vi "Read older Metadata channels.vi"(1 "Number of Channels":i32) -> (0 "Initial Info Cluster":T1[](array[typedef]))   [LabVIEW 2022 SP3]
uses:
  Controls/Initial Info Cluster.ctl
  Globals/Meas_global.vi
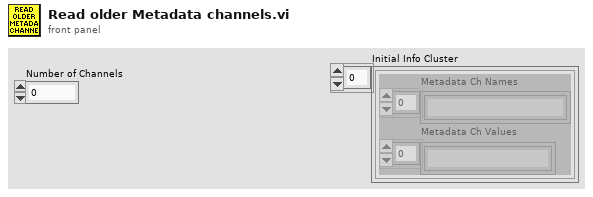
[diagram p1: front panel]
types:
  T1 = typedef "Initial Info Cluster.ctl" = cluster{"Metadata Ch Names":string[], "Metadata Ch Values":string[]}
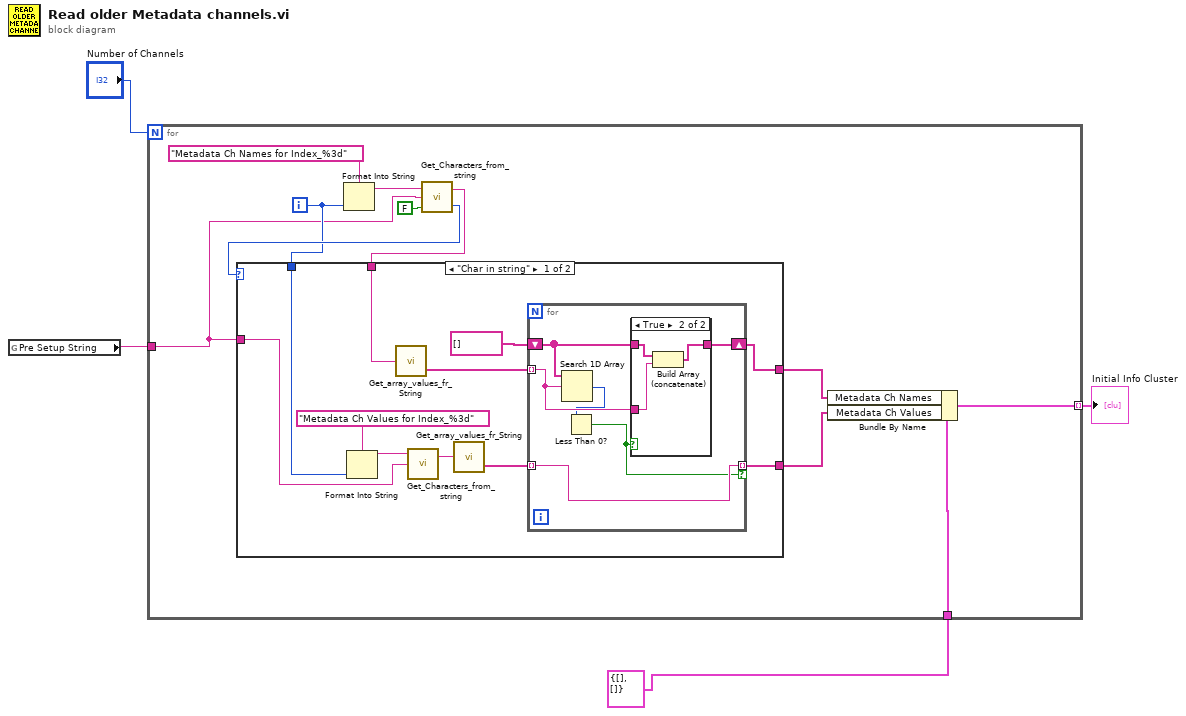
[diagram p0: block diagram]
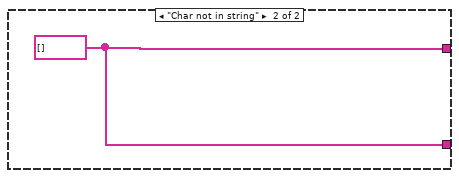
[diagram p3: hidden frame]
diagram:
  n1 = global read "Meas_global.vi" "Pre Setup String"() -> (w3:string)
  n2 = for {
    N: "Number of Channels" -> [_]
    tunnel: w3 -> [w9]
    tunnel: T1 {"Metadata Ch Names"=[], "Metadata Ch Values"=[]} ("Cluster") -> [w6]
    tunnel: [w5] -> w1 mode=indexing
    i -> [w11]
    n3 = Format Into String(format string="Metadata Ch Names for Index_%3d", w11) -> (resulting string=w13:string)  [unwired: 2 in, 1 out]
    n4 = call "Get_Characters_from_string.vi"("Show Dialog?"=FALSE, "Input string"=w9, "Variable name"=w13) -> ("Status"=w12:enum16{"Char in string", "Char not in string"}, "Value"=w10:string)
    n5 = case shown="\"Char in string\"" w12 {
      tunnel: w11 -> [w25 _]
      tunnel: w10 -> [w24 _]
      tunnel: [w18 w37] -> w8
      tunnel: [w17 w37] -> w7
      tunnel: w9 -> [w22 _]
      frame "Char in string" {
        n6 = Format Into String(format string="Metadata Ch Values for Index_%3d", w25) -> (resulting string=w23:string)  [unwired: 2 in, 1 out]
        n7 = call "Get_array_values_fr_String.vi"("String Value"=w24) -> ("String array"=w19:string[])  [unwired: 1 out]
        n8 = call "Get_Characters_from_string.vi"("Input string"=w22, "Variable name"=w23) -> ("Value"=w21:string)  [unwired: 1 in, 1 out]
        n9 = call "Get_array_values_fr_String.vi"("String Value"=w21) -> ("String array"=w16:string[])  [unwired: 1 out]
        n10 = for {
          shift-right: [w32] -> w18
          shift-left: string[] [] -> [w31]
          tunnel: w19 -> [w29] mode=indexing
          tunnel: [w30] -> w17 mode=indexing if=w27
          tunnel: w16 -> [w30] mode=indexing
          n11 = Search 1D Array(1D array=w31, element=w29) -> (index of element=w28:i32)  [unwired: 1 in]
          n12 = Less Than 0?(x=w28) -> (x < 0?=w27:bool)
          n13 = case shown="True" w27 {
            tunnel: w29 -> [_ w36]
            tunnel: [w33 w35] -> w32
            tunnel: w31 -> [w33 w34]
            frame False {
            }
            frame True {
              n14 = Build Array (concatenate)(w34, w36) -> (w35:string[])
            }
          }
        }
      }
      frame "Char not in string" {
        w37 = string[] [] ("String array")
      }
    }
    n15 = Bundle By Name(cluster=w6, "Metadata Ch Names"=w8, "Metadata Ch Values"=w7) -> (w5:T1)
  }
  "Initial Info Cluster" <- w1
